vi "Flatten.vi"(8 "error in (no error)":errorcluster, 11 "Reader in":refnum<class "Reader.lvclass">) -> (0 "error out":errorcluster, 3 "Reader out":refnum<class "Reader.lvclass">)   [LabVIEW 2015, in "Reader.lvclass"]
uses:
  Reader.lvclass
  Reader.lvclass/Reader.ctl
  Global/File Locations.vi
  <vilib>/Utility/xml.llb/Write to XML File(string).vi
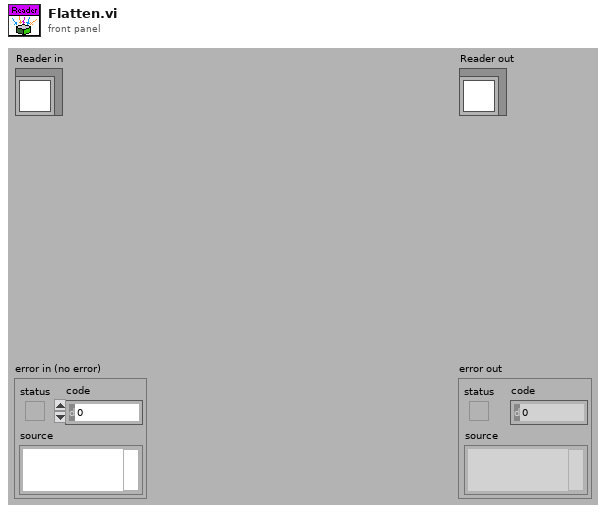
[diagram p1: front panel]
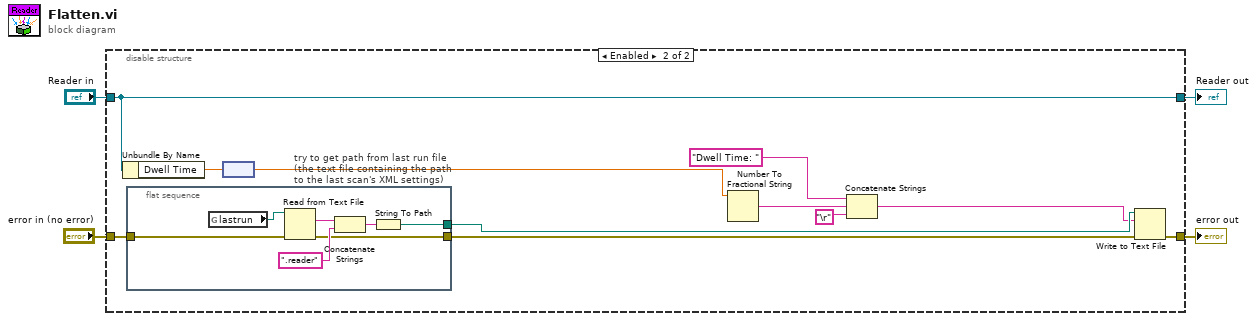
[diagram p0: block diagram]
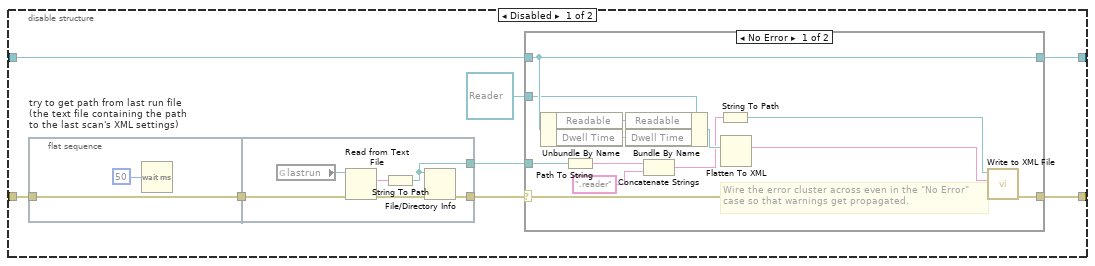
[diagram p2: hidden frame]
diagram:
  n1 = disable-structure shown="Enabled" {
    disable-tunnel: [w11 w44] -> w4
    disable-tunnel: "Reader in" -> [w10 w46]
    disable-tunnel: [w9 w46] -> w2
    disable-tunnel: "error in (no error)" -> [w7 w45]
    frame Disabled {
      n2 = flat-sequence "try to get path from last run file\n(the text file containing the path\nto the last scan's XML settings)" {
        tunnel: w7 -> [w14]
        tunnel: [w14] -> w12
        tunnel: [w20] -> w6
        tunnel: [w15] -> w5
        tunnel: w12 -> [w17]
        frame #0 {
          n3 = Wait (ms)(milliseconds to wait=u32 50) -> ()  [unwired: 1 out]
        }
        frame #1 {
          n4 = global read "File Locations.vi" "lastrun"() -> (w18:path)
          n5 = Read from Text File(file (use dialog)=w18, error in=w17) -> (text=w19:string, error out=w16:errorcluster)  [unwired: 4 out]
          n6 = String To Path(string=w19) -> (path=w20:path)
          n7 = File/Directory Info(path=w20, error in=w16) -> (error out=w15:errorcluster)  [unwired: 6 out]
        }
      }
      n8 = case shown="No Error" w5 {
        selector: w5 -> [w26 w35]
        tunnel: [w25 w35] -> w11
        tunnel: [w33 w34] -> w9
        tunnel: w10 -> [w33 w34]
        tunnel: refnum<class "Reader.lvclass"> refnum ("Reader.lvclass") -> [w31 _]
        tunnel: w6 -> [w24 _]
        frame No Error {
          # "Wire the error cluster across even in the \"No Error\"\ncase so that warnings get propagated."
          n9 = Unbundle By Name(w33) -> ("Readable"=w30:refnum<class "Readable.lvclass">, "Dwell Time"=w29:dbl[unit])
          n10 = Path To String(path=w24) -> (string=w23:string)
          n11 = Bundle By Name(cluster=w31, "Readable"=w30, "Dwell Time"=w29) -> (w28:refnum<class "Reader.lvclass">)
          n12 = Concatenate Strings(w23, ".reader") -> (w22:string)
          n13 = String To Path(string=w22) -> (path=w21:path)
          n14 = Flatten To XML(anything=w28) -> (xml string=w27:string)
          n15 = call-poly <vilib>:"Write to XML File.vi"("error in (no error)"=w26, "XML Input"=w27, "XML File Path"=w21) -> ("error out"=w25:errorcluster)  [unwired: 6 in, 2 out]
        }
        frame Error {
        }
      }
    }
    frame Enabled {
      n16 = Unbundle By Name(w46) -> ("Dwell Time"=w41:dbl[unit])
      n17 = flat-sequence "try to get path from last run file\n(the text file containing the path\nto the last scan's XML settings)" {
        tunnel: [w53] -> w42
        tunnel: [w47] -> w43
        tunnel: w45 -> [w51]
        frame #0 {
          n18 = global read "File Locations.vi" "lastrun"() -> (w52:path)
          n19 = Read from Text File(file (use dialog)=w52, error in=w51) -> (text=w50:string, error out=w47:errorcluster)  [unwired: 4 out]
          n20 = Concatenate Strings(w50, ".reader") -> (w48:string)
          n21 = String To Path(string=w48) -> (path=w53:path)
        }
      }
      n22 = node(w41) -> (w36:dbl)
      n23 = Number To Fractional String(number=w36) -> (F-format string=w40:string)  [unwired: 3 in]
      n24 = Concatenate Strings("Dwell Time: ", w40, "\r") -> (w37:string)
      n25 = Write to Text File(file (use dialog)=w42, text=w37, error in=w43) -> (error out=w44:errorcluster)  [unwired: 1 in, 2 out]
    }
  }
  "error out" <- w4
  "Reader out" <- w2
